vi "niRFUtil RFHS Channelizer ProcessCPUContext.vi"(0 "CPU Context":string) -> (4 "Exec Config":T1 {"CPU Context" format="%.0x"})   [LabVIEW 2015, in "niRFUtil.lvlib"]
uses:
  niRFUtil.lvlib
  Includes/niRFUtil RFHS Channelizer CPUInfo.ctl
  Utilities/niRFUtil RFHS Util CPU Context.ctl
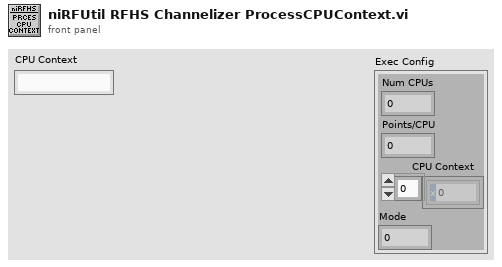
[diagram p1: front panel]
types:
  T1 = typedef "niRFUtil.lvlib/niRFUtil RFHS Channelizer CPUInfo.ctl" = cluster{"Num CPUs":u32, "Points/CPU":u32, "CPU Context":T2, "Mode":i32}
  T2 = typedef "niRFUtil.lvlib/niRFUtil RFHS Util CPU Context.ctl" = u64[]
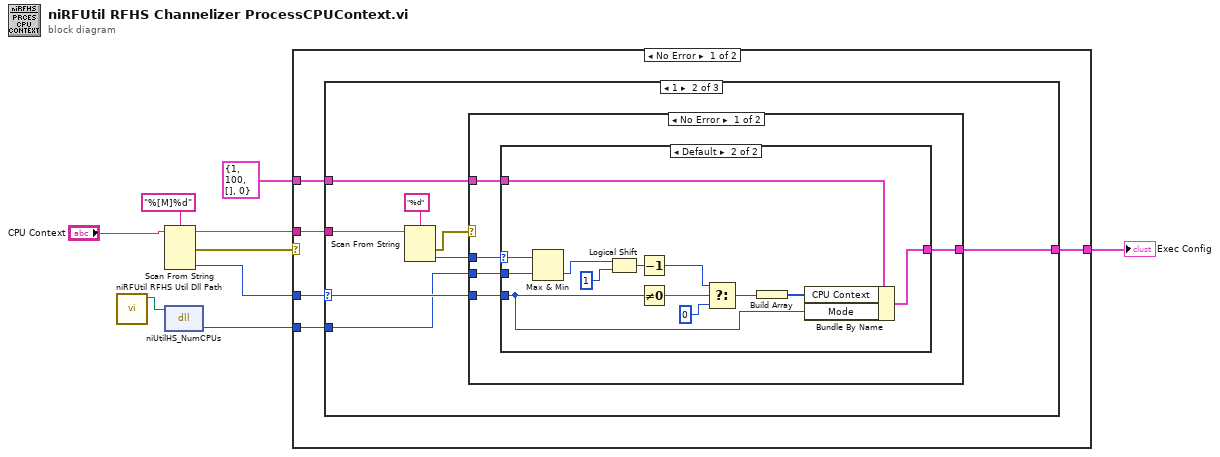
[diagram p0: block diagram]
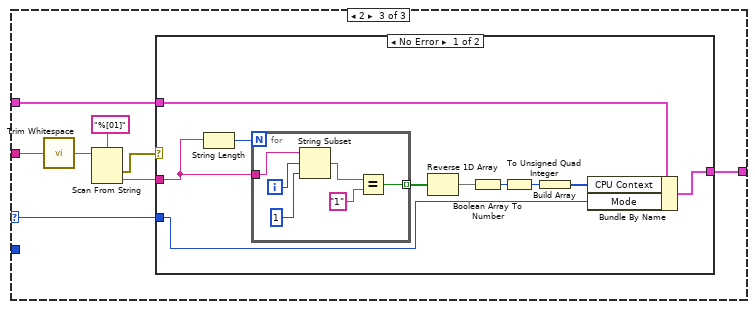
[diagram p5: hidden frame]
diagram:
  n1 = call "niRFUtil RFHS Util Dll Path.vi"() -> ("Path"=w2:path)  [unwired: 7 in, 4 out]
  n2 = Scan From String(format string="%[M]%d", input string="CPU Context") -> (remaining string=w3:string, error out=w4:errorcluster, output 2=w5:i32)  [unwired: 5 in, 1 out]
  n3 = dll-call lib="?" fn="niUtilHS_NumCPUs"(path in=w2) -> ("return type"=w1:i32)  [unwired: 2 in, 2 out]
  n4 = case shown="No Error" w4 {
    tunnel: [w14 w69] -> w8
    tunnel: T1 {"Num CPUs"=1, "Points/CPU"=100, "CPU Context"=[], "Mode"=0} ("Exec Config") -> [w13 w69]
    tunnel: w5 -> [w12 _]
    tunnel: w3 -> [w11 _]
    tunnel: w1 -> [w10 _]
    frame No Error {
      n5 = case shown="1" w12 {
        selector: w12 -> [_ w18 w46]
        tunnel: [w15 w23 w51] -> w14
        tunnel: w13 -> [w15 w22 w50]
        tunnel: w11 -> [_ w21 w49]
        tunnel: w10 -> [_ w16 _]
        frame Default {
        }
        frame 1 {
          n6 = Scan From String(format string="%d", input string=w21) -> (error out=w17:errorcluster, output 1=w19:i32)  [unwired: 3 in, 2 out]
          n7 = case shown="No Error" w17 {
            tunnel: [w28 w43] -> w23
            tunnel: w22 -> [w27 w43]
            tunnel: w19 -> [w26 _]
            tunnel: w18 -> [w25 _]
            tunnel: w16 -> [w24 _]
            frame No Error {
              n8 = case shown="Default" w26 {
                selector: w26 -> [_ w33]
                tunnel: [w29 w42] -> w28
                tunnel: w27 -> [w29 w30]
                tunnel: w25 -> [_ w34]
                tunnel: w24 -> [_ w32]
                frame 0 {
                }
                frame Default {
                  n9 = Max & Min(x=w33, y=w32) -> (min(x,y)=w31:i32)  [unwired: 1 out]
                  n10 = Logical Shift(y=w31, x=u64 1) -> (x << y=w38:u64)
                  n11 = Decrement(x=w38) -> (x-1=w37:u64)
                  n12 = Not Equal To 0?(x=w34) -> (x != 0?=w41:bool)
                  n13 = Select(t=w37, s=w41, f=u32 0) -> (s? t:f=w36:u64)
                  n14 = Build Array(w36) -> (w35:u64[])
                  n15 = Bundle By Name(cluster=w30, "CPU Context"=w35, "Mode"=w34) -> (w42:T1)
                }
              }
            }
            frame Error {
            }
          }
        }
        frame 2 {
          n16 = call <vilib>:"Trim Whitespace.vi"("string"=w49) -> ("trimmed string"=w44:string)  [unwired: 1 in]
          n17 = Scan From String(format string="%[01]", input string=w44) -> (error out=w45:errorcluster, output 1=w47:string)  [unwired: 3 in, 2 out]
          n18 = case shown="No Error" w45 {
            tunnel: [w61 w68] -> w51
            tunnel: w50 -> [w60 w68]
            tunnel: w47 -> [w56 _]
            tunnel: w46 -> [w59 _]
            frame No Error {
              n19 = String Length(string=w56) -> (length=w57:i32)
              n20 = for {
                N: w57 -> [_]
                tunnel: w56 -> [w67]
                tunnel: [w64] -> w55 mode=indexing
                i -> [w66]
                n21 = String Subset(string=w67, offset (0)=w66, length (rest)=1 ("length (rest)")) -> (substring=w63:string)
                n22 = Equal?(x=w63, y="1" ("x")) -> (x = y?=w64:bool)
              }
              n23 = Reverse 1D Array(array=w55) -> (reversed array=w52:bool[])
              n24 = Boolean Array To Number(Boolean array=w52) -> (number=w54:u32)
              n25 = To Unsigned Quad Integer(1:w54) -> (0:w53:u64)
              n26 = Build Array(w53) -> (w58:u64[])
              n27 = Bundle By Name(cluster=w60, "CPU Context"=w58, "Mode"=w59) -> (w61:T1)
            }
            frame Error {
            }
          }
        }
      }
    }
    frame Error {
    }
  }
  "Exec Config" <- w8
